vi "sio flush.vi"(10 "func":i32, 11 "port":i32) -> (2 "Status":i32, 3 "port out":i32)   [LabVIEW 2015, in "PCOMM.lvlib"]
doc: "int WINAPI sio_flush(int port, int func);"
uses:
  PCOMM.lvlib
  PCOMM.DLL
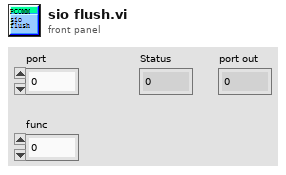
[diagram p1: front panel]
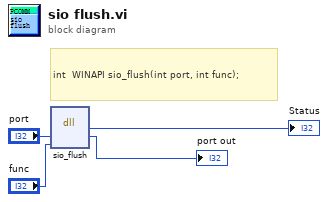
[diagram p0: block diagram]
diagram:
  # "int  WINAPI sio_flush(int port, int func);"
  n1 = dll-call lib="PTH2^abs EDesktopLabview串口助手串口助手2.0Ing10_v3.2.0SubVIpcomm库PCOMM.*" fn="sio_flush"("port"="port", "func"="func") -> (→"Status":i32, "port"=→"port out":i32)  [unwired: 4 in, 2 out]
